vi "Close.vi"(8 "error in (no error)":errorcluster, 11 "DAQmx Base CFG in":refnum<class "DAQmx Base CFG.lvclass">) -> (0 "error out":errorcluster, 3 "DAQmx Base CFG out":refnum<class "DAQmx Base CFG.lvclass">)   [LabVIEW 2023, in "DAQmx Base CFG.lvclass"]
uses:
  DAQmx Base CFG.lvclass
  DAQmx Base CFG.lvclass/DAQmx Base CFG.ctl
  Configuration/Configuration Semaphore/CFG Semaphore.lvclass
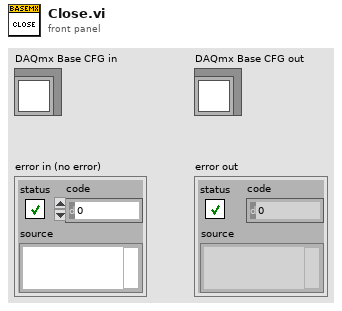
[diagram p1: front panel]
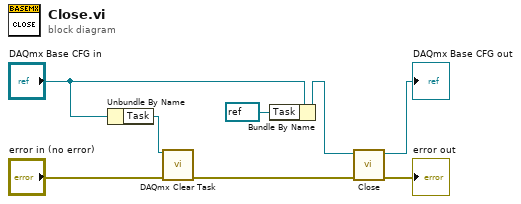
[diagram p0: block diagram]
diagram:
  n1 = Unbundle By Name("DAQmx Base CFG in") -> ("Task"=w8:refnum<k21>)
  n2 = call <vilib>:"DAQmx Clear Task.vi"("task in"=w8, "error in"="error in (no error)") -> ("error out"=w4:errorcluster)  [unwired: 13 in]
  n3 = Bundle By Name(cluster="DAQmx Base CFG in", "Task"=refnum<k21> refnum) -> (w2:refnum<class "DAQmx Base CFG.lvclass">)
  n4 = call-parent "Close.vi"("error in (no error)"=w4, "CFG Semaphore in"=w2) -> ("error out"=→"error out":errorcluster, "CFG Semaphore out"=→"DAQmx Base CFG out":refnum<class "DAQmx Base CFG.lvclass">)  [unwired: 8 in]
